vi "_builtins_select_controls.vi"(8 "error in (no error)":errorcluster, 9 "Selection":T1, 10 "Focus":enum8{"FP", "BD"}(ring), 11 "VI Refnum in":refnum<vi>) -> (0 "error out":errorcluster, 3 "VI Refnum out":refnum<vi>)   [LabVIEW 2019, in "Script.lvlib"]
doc: "On the Panel, makes a new selection of Controls, Indicators or Both.\nOn the Diagram, makes a new selection of Control Terminals, Indicator Terminals or Both.\n\nCreated by: Ryan Pacini"
uses:
  Script.lvlib
  _builtins_selection.ctl
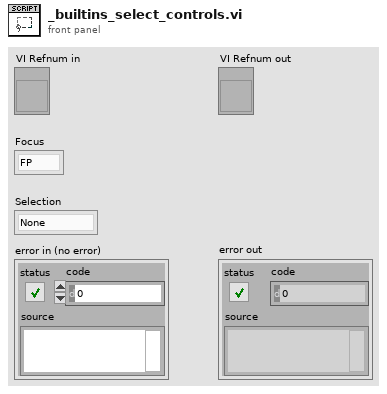
[diagram p1: front panel]
types:
  T1 = typedef "Script.lvlib/_builtins_selection.ctl" = enum8{"None", "Controls", "Indicators", "Both"}
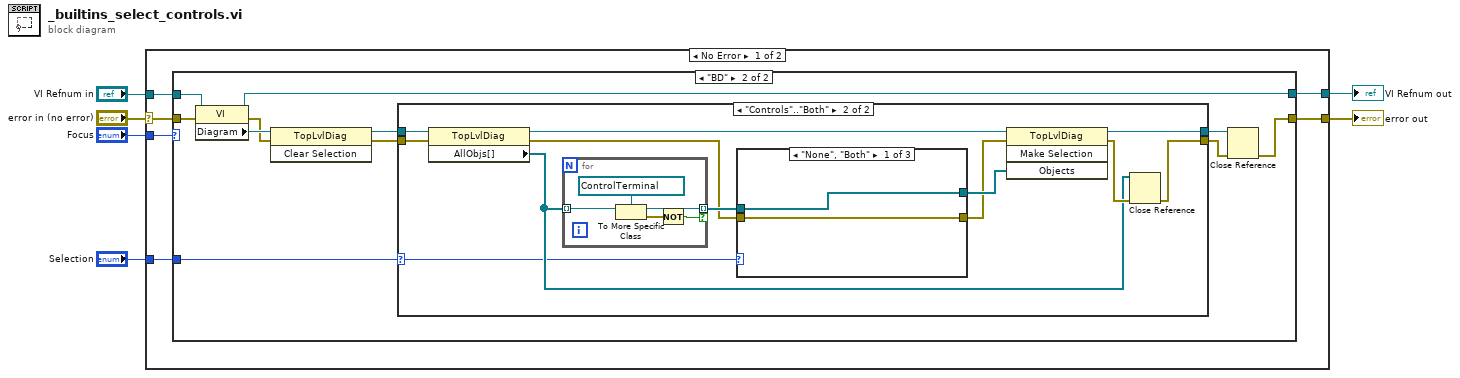
[diagram p0: block diagram]
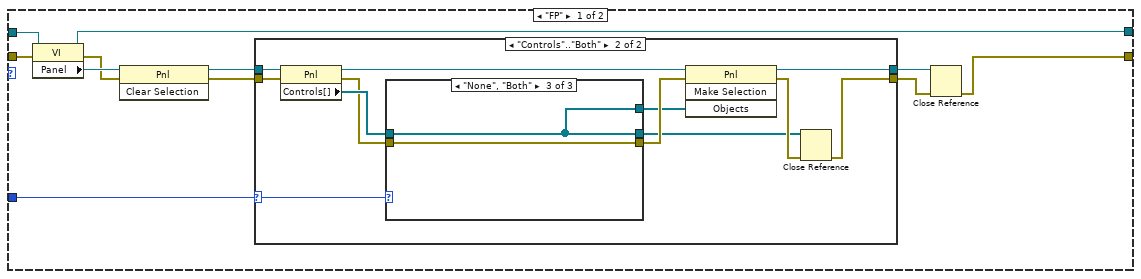
[diagram p2: hidden frame]
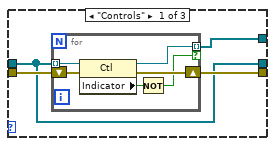
[diagram p4: hidden frame]
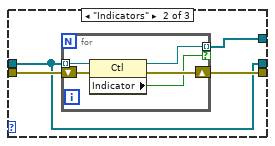
[diagram p5: hidden frame]
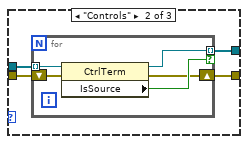
[diagram p7: hidden frame]
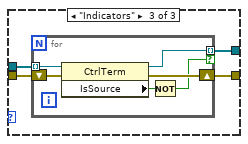
[diagram p8: hidden frame]
diagram:
  n1 = case shown="No Error" "error in (no error)" {
    selector: "error in (no error)" -> [w9 w110]
    tunnel: "Focus" -> [w12 _]
    tunnel: "Selection" -> [w11 _]
    tunnel: "VI Refnum in" -> [w10 w111]
    tunnel: [w8 w110] -> w2
    tunnel: [w7 w111] -> w1
    frame No Error {
      n2 = case shown="\"BD\"" w12 {
        tunnel: w9 -> [w23 w69]
        tunnel: w10 -> [w22 w68]
        tunnel: w11 -> [w19 w59]
        tunnel: [w17 w64] -> w8
        tunnel: [w13 w63] -> w7
        frame "FP" {
          n3 = property class="VI"(reference=w22, error in=w23) -> (reference out=w13:refnum<vi>, error out=w15:errorcluster, "Panel"=w21:refnum<vi>)
          n4 = invoke class="Pnl" method="Clear Selection"(reference=w21, error in=w15) -> (reference out=w16:refnum<vi>, error out=w14:errorcluster)  [unwired: 1 in, 1 out]
          n5 = case shown="\"Controls\"..\"Both\"" w19 {
            selector: w19 -> [_ w31]
            tunnel: [w25 w32] -> w20
            tunnel: [w24 w28] -> w18
            tunnel: w16 -> [w25 w27]
            tunnel: w14 -> [w24 w26]
            frame "None" {
            }
            frame "Controls".."Both" {
              n6 = property class="Pnl"(reference=w27, error in=w26) -> (reference out=w35:refnum<vi>, error out=w36:errorcluster, "Controls[]"=w37:refnum<vi>[])
              n7 = case shown="\"None\", \"Both\"" w31 {
                tunnel: w37 -> [w38 w48 w58]
                tunnel: w36 -> [w41 w51 w57]
                tunnel: [w40 w50 w57] -> w34
                tunnel: [w39 w49 w58] -> w33
                tunnel: [w38 w48 w58] -> w29
                frame "Controls" {
                  n8 = for {
                    tunnel: w38 -> [w47] mode=indexing
                    tunnel: [w45] -> w39 mode=indexing if=w42
                    shift-right: [w43] -> w40
                    shift-left: w41 -> [w46]
                    n9 = property class="Ctl"(reference=w47, error in=w46) -> (reference out=w45:refnum<vi>, error out=w43:errorcluster, "Indicator"=w44:bool)
                    n10 = Not(x=w44) -> (.not. x?=w42:bool)
                  }
                }
                frame "Indicators" {
                  n11 = for {
                    tunnel: w48 -> [w56] mode=indexing
                    tunnel: [w54] -> w49 mode=indexing if=w52
                    shift-right: [w53] -> w50
                    shift-left: w51 -> [w55]
                    n12 = property class="Ctl"(reference=w56, error in=w55) -> (reference out=w54:refnum<vi>, error out=w53:errorcluster, "Indicator"=w52:bool)
                  }
                }
                frame "None", "Both" {
                }
              }
              n13 = invoke class="Pnl" method="Make Selection"(reference=w35, error in=w34, "Objects"=w33) -> (reference out=w32:refnum<vi>, error out=w30:errorcluster)  [unwired: 1 in, 2 out]
              n14 = Close Reference(reference=w29, error in (no error)=w30) -> (error out=w28:errorcluster)
            }
          }
          n15 = Close Reference(reference=w20, error in (no error)=w18) -> (error out=w17:errorcluster)
        }
        frame "BD" {
          n16 = property class="VI"(reference=w68, error in=w69) -> (reference out=w63:refnum<vi>, error out=w61:errorcluster, "Diagram"=w67:refnum<vi>)
          n17 = invoke class="TopLvlDiag" method="Clear Selection"(reference=w67, error in=w61) -> (reference out=w62:refnum<vi>, error out=w60:errorcluster)  [unwired: 1 in, 1 out]
          n18 = case shown="\"Controls\"..\"Both\"" w59 {
            selector: w59 -> [_ w72]
            tunnel: [w70 w82] -> w66
            tunnel: [w71 w79] -> w65
            tunnel: w62 -> [w70 w78]
            tunnel: w60 -> [w71 w77]
            frame "None" {
            }
            frame "Controls".."Both" {
              n19 = property class="TopLvlDiag"(reference=w78, error in=w77) -> (reference out=w83:refnum<vi>, error out=w74:errorcluster, "AllObjs[]"=w80:refnum<vi>[])
              n20 = for {
                tunnel: w80 -> [w109] mode=indexing
                tunnel: [w107] -> w76 mode=indexing if=w105
                n21 = To More Specific Class(target class=refnum<vi> refnum, reference=w109) -> (specific class reference=w107:refnum<vi>, error out=w106:errorcluster)  [unwired: 1 in]
                n22 = Not(x=w106) -> (.not. x?=w105:bool)
              }
              n23 = case shown="\"None\", \"Both\"" w72 {
                tunnel: w76 -> [w84 w89 w98]
                tunnel: [w84 w88 w97] -> w75
                tunnel: w74 -> [w85 w87 w96]
                tunnel: [w85 w86 w95] -> w73
                frame "None", "Both" {
                }
                frame "Controls" {
                  n24 = for {
                    tunnel: w89 -> [w94] mode=indexing
                    tunnel: [w93] -> w88 mode=indexing if=w92
                    shift-right: [w90] -> w86
                    shift-left: w87 -> [w91]
                    n25 = property class="CtrlTerm"(reference=w94, error in=w91) -> (reference out=w93:refnum<vi>, error out=w90:errorcluster, "IsSource"=w92:bool)
                  }
                }
                frame "Indicators" {
                  n26 = for {
                    tunnel: w98 -> [w104] mode=indexing
                    tunnel: [w103] -> w97 mode=indexing if=w99
                    shift-right: [w100] -> w95
                    shift-left: w96 -> [w101]
                    n27 = property class="CtrlTerm"(reference=w104, error in=w101) -> (reference out=w103:refnum<vi>, error out=w100:errorcluster, "IsSource"=w102:bool)
                    n28 = Not(x=w102) -> (.not. x?=w99:bool)
                  }
                }
              }
              n29 = invoke class="TopLvlDiag" method="Make Selection"(reference=w83, error in=w73, "Objects"=w75) -> (reference out=w82:refnum<vi>, error out=w81:errorcluster)  [unwired: 1 in, 2 out]
              n30 = Close Reference(reference=w80, error in (no error)=w81) -> (error out=w79:errorcluster)
            }
          }
          n31 = Close Reference(reference=w66, error in (no error)=w65) -> (error out=w64:errorcluster)
        }
      }
    }
    frame Error {
    }
  }
  "VI Refnum out" <- w1
  "error out" <- w2
